vi "IntakeUpdateSpeeds.vi"(9 "IntakeLeftRollerSpeed":dbl, 10 "IntakeRightRollerSpeed":dbl) -> ()   [LabVIEW 2014, in "IntakeLib.lvlib"]
uses:
  IntakeLib.lvlib
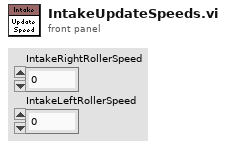
[diagram p1: front panel]
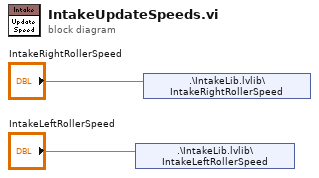
[diagram p0: block diagram]
diagram:
  n1 = shared-variable ".\\IntakeLib.lvlib\\IntakeLeftRollerSpeed"("IntakeLeftRollerSpeed") -> ()  [unwired: 1 in, 1 out]
  n2 = shared-variable ".\\IntakeLib.lvlib\\IntakeRightRollerSpeed"("IntakeRightRollerSpeed") -> ()  [unwired: 1 in, 1 out]
